vi "Map STUFF.vi"(7 "Type Name Library File Path in":T2, 9 "Implemented Class File Paths":path[](array[path]), 10 "Type":T1) -> (5 "Type Name Library File Path out":T2)   [LabVIEW 2020, in "_Shared.lvlib"]
uses:
  _Shared.lvlib
  Name Library File Path.ctl
  Type.ctl
  Type Name Library File Path.ctl
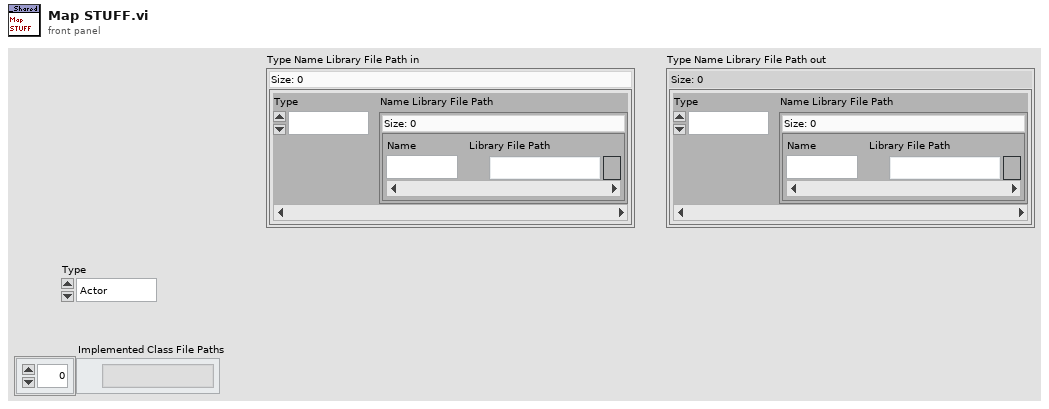
[diagram p1: front panel]
types:
  T1 = typedef "_Shared.lvlib/Type.ctl" = enum16{"Actor", "Msg"}
  T2 = typedef "_Shared.lvlib/Type Name Library File Path.ctl" = map{T1, T3}
  T3 = typedef "_Shared.lvlib/Name Library File Path.ctl" = map{string, path}
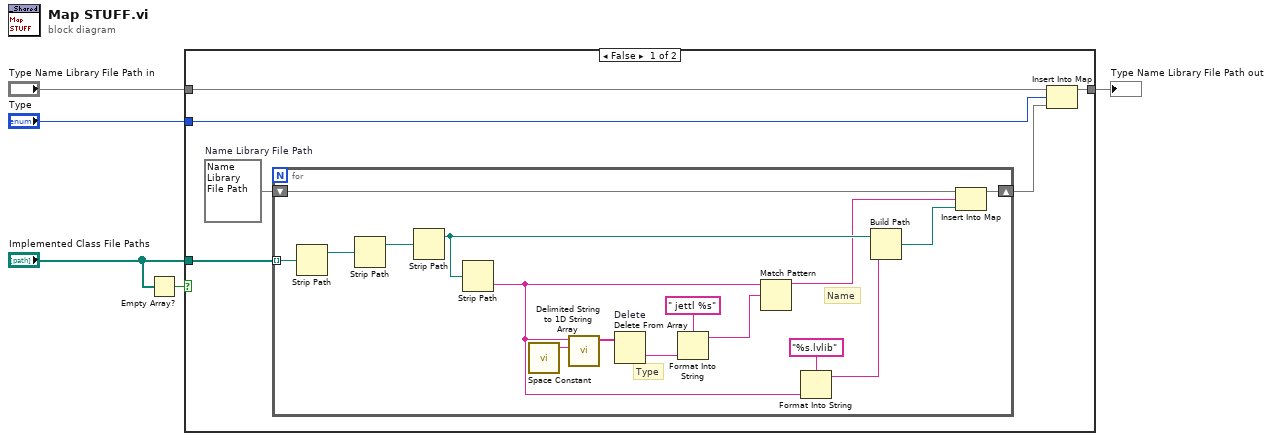
[diagram p0: block diagram]
diagram:
  n1 = Empty Array?(array="Implemented Class File Paths") -> (empty?=w1:bool)
  n2 = case shown="False" w1 {
    tunnel: "Type Name Library File Path in" -> [w11 w28]
    tunnel: [w10 w28] -> w4
    tunnel: "Type" -> [w9 _]
    tunnel: "Implemented Class File Paths" -> [w6 _]
    frame False {
      w8 = T3 {}  # Name Library File Path
      n3 = for {
        tunnel: w6 -> [w23] mode=indexing
        shift-right: [w26] -> w7
        shift-left: w8 -> [w27]
        # "Name"
        # "Type"
        n4 = Strip Path(path=w23) -> (stripped path=w25:path)  [unwired: 1 out]
        n5 = Strip Path(path=w25) -> (stripped path=w24:path)  [unwired: 1 out]
        n6 = Strip Path(path=w24) -> (stripped path=w18:path)  [unwired: 1 out]
        n7 = Strip Path(path=w18) -> (name=w14:string)  [unwired: 1 out]
        n8 = call <vilib>:"Space Constant.vi"() -> ("String"=w22:string)
        n9 = call <vilib>:"Delimited String to 1D String Array.vi"("delimiter"=w22, "delimited string"=w14) -> ("string array"=w21:string[])  [unwired: 9 in]
        n10 = Delete From Array "Delete"(array=w21) -> (deleted portion=w17:string)  [unwired: 2 in, 1 out]
        n11 = Format Into String(format string=" jettl %s", w17) -> (resulting string=w15:string)  [unwired: 2 in, 1 out]
        n12 = Match Pattern(string=w14, regular expression=w15) -> (before substring=w13:string)  [unwired: 1 in, 3 out]
        n13 = Format Into String(format string="%s.lvlib", w14) -> (resulting string=w12:string)  [unwired: 2 in, 1 out]
        n14 = Build Path(base path=w18, name or relative path=w12) -> (appended path=w19:path)
        n15 = Insert Into Map(map in=w27, key=w13, value=w19) -> (map out=w26:T3)  [unwired: 2 out]
      }
      n16 = Insert Into Map(map in=w11, key=w9, value=w7) -> (map out=w10:T2)  [unwired: 2 out]
    }
    frame True {
    }
  }
  "Type Name Library File Path out" <- w4
